vi "GeneratorUI-Advanced.vi"(8 "error in":errorcluster, 9 "Unattended Mode":bool, 10 "File configurations":T1(array[cluster]), 11 "Top level output path":path) -> (0 "error out":errorcluster)   [LabVIEW 2017]
uses:
  PathConfiguration.vi
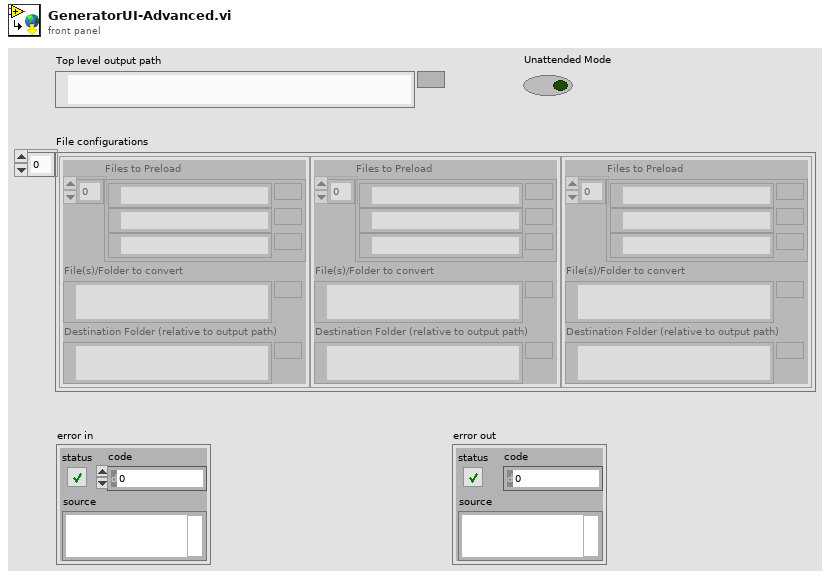
[diagram p1: front panel]
types:
  T1 = cluster{"Files to Preload":path[], "File(s)/Folder to convert":path, "Destination Folder (relative to output path)":path}[]
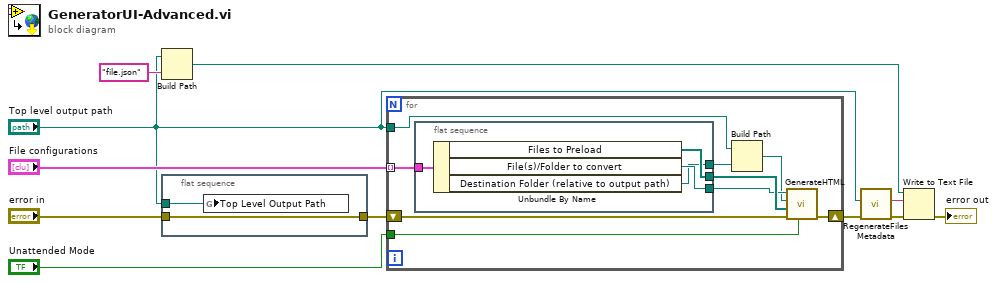
[diagram p0: block diagram]
diagram:
  n1 = Build Path(base path="Top level output path", name or relative path="file.json") -> (appended path=w8:path)
  n2 = flat-sequence {
    tunnel: "Top level output path" -> [w13]
    tunnel: "error in" -> [w12]
    tunnel: [w12] -> w1
    frame #0 {
      n3 = global write "PathConfiguration.vi" "Top Level Output Path"(w13) -> ()
    }
  }
  n4 = for {
    tunnel: "File configurations" -> [w22] mode=indexing
    shift-right: [w15] -> w9
    shift-left: w1 -> [w19]
    tunnel: "Top level output path" -> [w18]
    tunnel: "Unattended Mode" -> [w14]
    n5 = flat-sequence {
      tunnel: w22 -> [w26]
      tunnel: [w25] -> w21
      tunnel: [w24] -> w20
      tunnel: [w23] -> w16
      frame #0 {
        n6 = Unbundle By Name(w26) -> ("Files to Preload"=w25:path[], "File(s)/Folder to convert"=w24:path, "Destination Folder (relative to output path)"=w23:path)
      }
    }
    n7 = Build Path(base path=w18, name or relative path=w16) -> (appended path=w17:path)
    n8 = call "GenerateHTML.vi"("Unattended Mode"=w14, "error in (no error)"=w19, "Files to preload"=w21, "Destination Directory"=w17, "Source directory/files"=w20) -> ("error out"=w15:errorcluster)  [unwired: 5 in, 1 out]
  }
  n9 = call "RegenerateFilesMetadata.vi"("error in (no error)"=w9, "Path"="Top level output path") -> ("error out"=w6:errorcluster, "String"=w7:string)  [unwired: 7 in, 1 out]
  n10 = Write to Text File(file (use dialog)=w8, text=w7, error in=w6) -> (error out=→"error out":errorcluster)  [unwired: 1 in, 2 out]
